vi "Search Replace UID String.vi"(7 "Replace All Numeric Inputs":bool, 10 "UID":i32, 11 "Input String":string) -> (3 "Output String":string)   [LabVIEW 2015, in "Front Panel Publisher.lvlib"]
doc: "This VI will search for UID%d or UID=%d in the Input String and replace it with the UID provided. Optionally all %d inputs can be replaced with this UID."
uses:
  Front Panel Publisher.lvlib
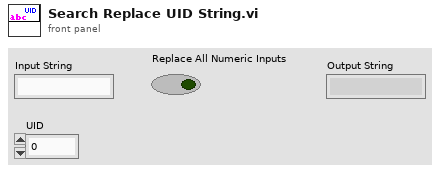
[diagram p1: front panel]
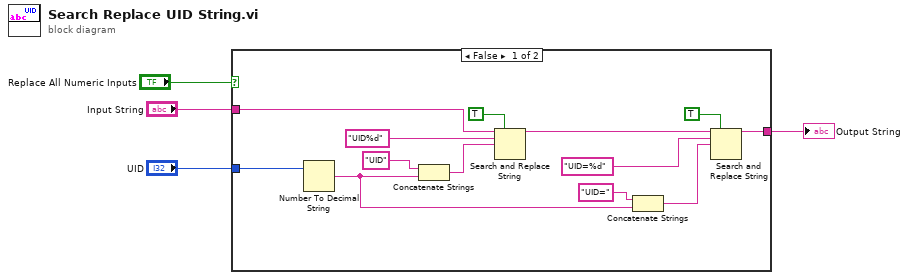
[diagram p0: block diagram]
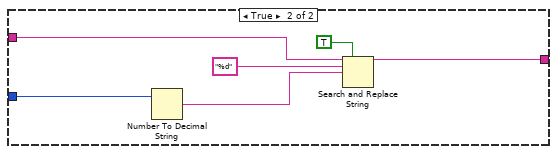
[diagram p2: hidden frame]
diagram:
  n1 = case shown="False" "Replace All Numeric Inputs" {
    tunnel: "UID" -> [w16 w21]
    tunnel: "Input String" -> [w14 w19]
    tunnel: [w5 w18] -> w2
    frame False {
      n2 = Number To Decimal String(number=w16) -> (decimal integer string=w7:string)  [unwired: 1 in]
      n3 = Concatenate Strings("UID" ("string"), w7) -> (w11:string)
      n4 = Search and Replace String(replace all?=TRUE ("replace all? (F)"), input string=w14, search string="UID%d", replace string=w11) -> (result string=w12:string)  [unwired: 4 in, 3 out]
      n5 = Concatenate Strings("UID=" ("string"), w7) -> (w6:string)
      n6 = Search and Replace String(replace all?=TRUE ("replace all? (F)"), input string=w12, search string="UID=%d", replace string=w6) -> (result string=w5:string)  [unwired: 4 in, 3 out]
    }
    frame True {
      n7 = Number To Decimal String(number=w21) -> (decimal integer string=w20:string)  [unwired: 1 in]
      n8 = Search and Replace String(replace all?=TRUE ("replace all? (F)"), input string=w19, search string="%d", replace string=w20) -> (result string=w18:string)  [unwired: 4 in, 3 out]
    }
  }
  "Output String" <- w2
